vi "GOOP_LVClass_CreateNewWizard_Invoke.vi"(10 "New Item Parent":T1, 11 "Wizard":u64) -> (3 "Canceled":bool)   [LabVIEW 2020]
uses:
  <resource>/Framework/Providers/API/mxLvNIIM.ctl
  <resource>/Framework/Providers/Open_GDS/ClassProviders/Provider_EndevoGOOP300/GOOP300_SubVIs/GOOP300_MethodScopeType.ctl
  <resource>/Framework/Providers/Open_GDS/SubVIs/GOOP_ClassProviderClassType.ctl
  <resource>/Framework/Providers/Open_GDS/ClassProviders/Provider_BaseClassInterface/ClassWriter_class/ClassWriter.lvclass
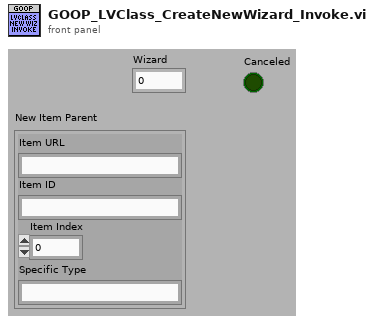
[diagram p1: front panel]
types:
  T1 = typedef "mxLvNIIM.ctl" = cluster{"Item URL":string, "Item ID":string, "Item Index":i32, "Specific Type":string}
  T2 = typedef "GOOP300_MethodScopeType.ctl" = enum16{"Use Parent Folder Scope", "Public", "Protected", "Private", "Community"}
  T3 = typedef "GOOP_ClassProviderClassType.ctl" = enum16{"ClassWriter", "ClassReader"}
  T4 = typedef "ClassWriter.lvclass/CreateClassData.ctl" = cluster{"ClassName":string, "ClassFolder":path, "ClassDescription":string, "ClassTemplateOptions":string, "BaseClass(ProjectStringPath or LvClassFilePath)":variant, "ExtraCreateParameters":variant, "FolderSuffix":string}
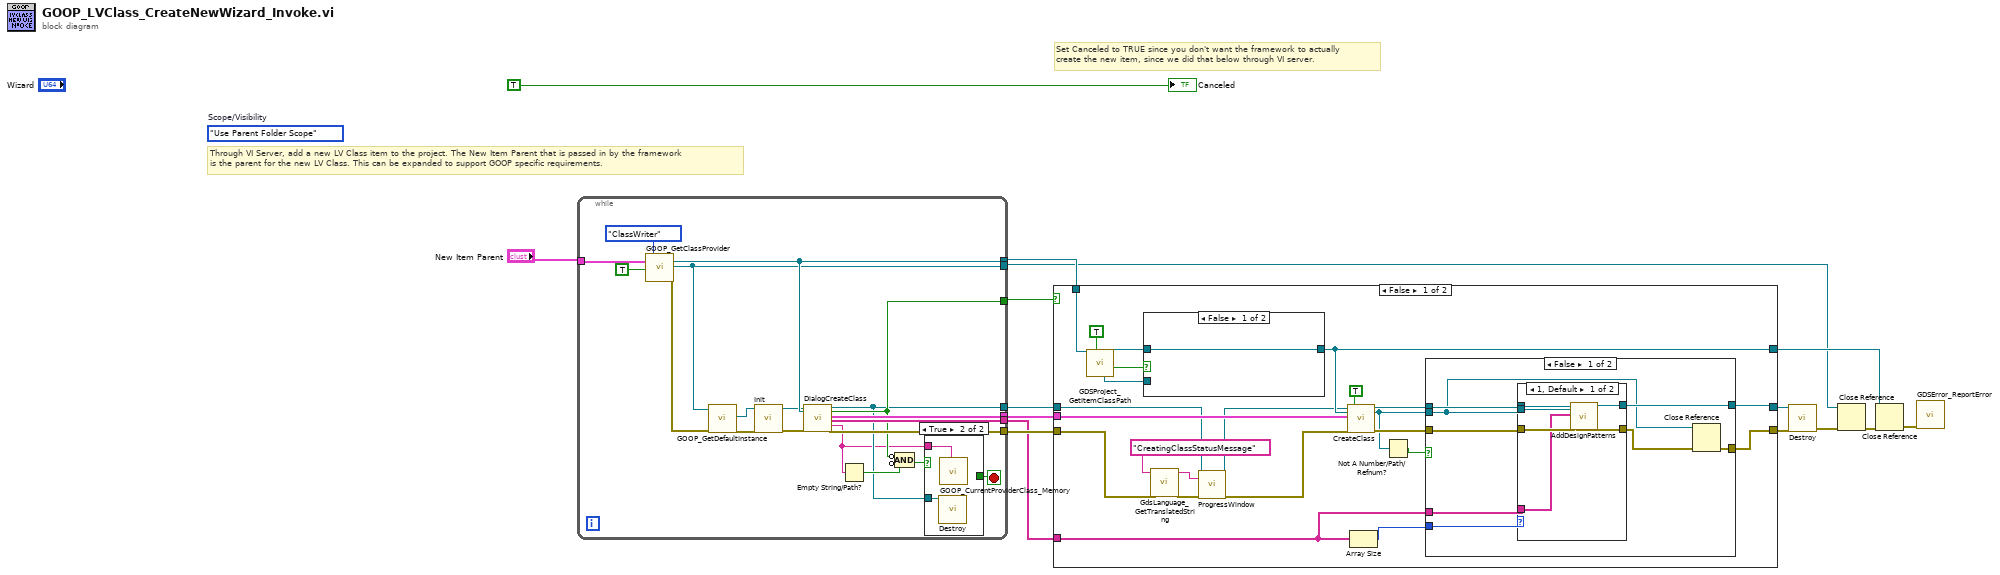
[diagram p0: block diagram]
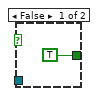
[diagram p2: hidden frame]
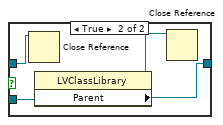
[diagram p5: hidden frame]
diagram:
  (unwired) GOOP300_MethodScopeType."Use Parent Folder Scope"  # Scope/Visibility
  # "Through VI Server, add a new LV Class item to the project. The New Item Parent that is passed in by the framework\nis the parent for the new LV Class. This can be expanded to support GOOP specific requirements."
  # "Set Canceled to TRUE since you don't want the framework to actually\ncreate the new item, since we did that below through VI server."
  n1 = while {
    tunnel: "New Item Parent" -> [w34]
    tunnel: [w17] -> w11
    tunnel: [w33] -> w10
    tunnel: [w32] -> w9
    tunnel: [w30] -> w6
    tunnel: [w25] -> w3
    tunnel: [w22] -> w2
    tunnel: [w21] -> w1
    stop <- w18 stop-if-true
    n2 = call <resource>:"GOOP_GetClassProvider.vi"("New Item Parent/Object"=w34, "CreateClass"=TRUE, "ProviderClassType"=GOOP_ClassProviderClassType."ClassWriter") -> ("ProjectItem"=w30:refnum<vi>, "LVClass.Open"=w25:refnum<vi>, "error out"=w24:errorcluster)  [unwired: 14 in]
    n3 = call <resource>:"GOOP_GetDefaultInstance.vi"("error in"=w24, "LVClassIn"=w25) -> ("error out"=w26:errorcluster, "ClassWriter.lvclass"=w23:refnum<class "ClassWriter.lvclass">)  [unwired: 7 in, 1 out]
    n4 = call-dynamic "Init.vi"("ClassWriter in"=w23, "error in (no error)"=w26) -> ("ClassWriter out"=w28:refnum<class "ClassWriter.lvclass">, "error out"=w27:errorcluster)  [unwired: 16 in]
    n5 = call-dynamic "DialogCreateClass.vi"("ClassWriter in"=w28, "ProjectItem Refnum"=w30, "error in (no error)"=w27) -> ("ClassWriter out"=w17:refnum<class "ClassWriter.lvclass">, "Cancelled"=w21:bool, "CreateClassData"=w32:T4, "DesignPatternsToAddAfterCreation"=w22:string[], "ChangeProviderRequested"=w16:string, "error out"=w33:errorcluster)  [unwired: 11 in]
    n6 = Empty String/Path?(string/path=w16) -> (empty?=w20:bool)
    n7 = Compound Arithmetic op=AND(invert w21, invert w20) -> (w19:bool)
    n8 = case shown="True" w19 {
      tunnel: w16 -> [_ w37]
      tunnel: [TRUE _] -> w18
      tunnel: w17 -> [_ w36]
      frame False {
      }
      frame True {
        n9 = call-dynamic "Destroy.vi"("ClassWriter.lvclass"=w36) -> ()  [unwired: 18 in, 1 out]
        n10 = call <resource>:"GOOP_CurrentProviderClass_Memory.vi"("SetDefaultClassProvider(Ignored if not wired)"=w37) -> ()  [unwired: 14 in, 5 out]
      }
    }
  }
  n11 = case shown="False" w1 {
    tunnel: [w40 w86] -> w14
    tunnel: [w48 w85] -> w13
    tunnel: w11 -> [w51 w86]
    tunnel: w10 -> [w45 w85]
    tunnel: w9 -> [w60 _]
    tunnel: w6 -> [w59 w84]
    tunnel: [w55 w84] -> w5
    tunnel: w2 -> [w44 _]
    frame False {
      n12 = call <resource>:"GDSProject_GetItemClassPath.vi"("ReturnRefToClass(False)"=TRUE, "ProjectItemRefIn"=w59) -> ("LvCLassFound"=w57:bool, "ProjectItemRefOut"=w56:refnum<vi>, "LvClassRef"=w54:refnum<vi>)  [unwired: 4 in, 3 out]
      n13 = case shown="False" w57 {
        tunnel: w56 -> [w79 w83]
        tunnel: [w79 w81] -> w55
        tunnel: w54 -> [_ w82]
        frame False {
        }
        frame True {
          n14 = Close Reference(reference=w83) -> ()  [unwired: 1 in, 1 out]
          n15 = property class="LVClassLibrary"(reference=w82) -> (reference out=w80:refnum<vi>, "Parent"=w81:refnum<vi>)  [unwired: 1 in, 1 out]
          n16 = Close Reference(reference=w80) -> ()  [unwired: 1 in, 1 out]
        }
      }
      n17 = call <resource>:"GdsLanguage_GetTranslatedString.vi"("StringID(s)"="CreatingClassStatusMessage" ("Message(Exit)"), "error in (no error)"=w45) -> ("FirstStringOut"=w53:string, "error out"=w46:errorcluster)  [unwired: 14 in, 2 out]
      n18 = call-dynamic "ProgressWindow.vi"("ClassWriter in"=w51, "Message(Exit)"=w53, "error in (no error)"=w46) -> ("ClassWriter out"=w50:refnum<class "ClassWriter.lvclass">, "error out"=w47:errorcluster)  [unwired: 15 in]
      n19 = call-dynamic "CreateClass.vi"("ClassWriter.lvclass"=w50, "ProjectTreePosition(String or Project Item Ref)"=w55, "CreateClassData"=w60, "error in (no error)"=w47, "KeepLvClassRefOpen(False)"=TRUE) -> ("ClassWriter.lvclass"=w42:refnum<class "ClassWriter.lvclass">, "LVClassLibraryRefnum"=w39:refnum<vi>, "error out"=w41:errorcluster)  [unwired: 11 in, 1 out]
      n20 = Array Size(array=w44) -> (size(s)=w43:i32)
      n21 = Not A Number/Path/Refnum?(number/path/refnum=w39) -> (NaN/Path/Refnum?=w38:bool)
      n22 = case shown="False" w38 {
        tunnel: [w68 w78] -> w48
        tunnel: w44 -> [w67 _]
        tunnel: w43 -> [w66 _]
        tunnel: w42 -> [w65 w77]
        tunnel: w41 -> [w64 w78]
        tunnel: [w63 w77] -> w40
        tunnel: w39 -> [w61 _]
        frame False {
          n23 = case shown="1, Default" w66 {
            tunnel: w65 -> [w74 w76]
            tunnel: w64 -> [w73 w75]
            tunnel: [w72 w75] -> w62
            tunnel: [w71 w76] -> w63
            tunnel: w67 -> [w70 _]
            tunnel: w61 -> [w69 _]
            frame 1, Default {
              n24 = call-dynamic "AddDesignPatterns.vi"("ClassWriterNative"=w74, "ClassItemRefIn"=w69, "DesignPatterns"=w70, "error in (no error)"=w73) -> ("ClassWriterNative"=w71:refnum<class "ClassWriter.lvclass">, "error out"=w72:errorcluster)  [unwired: 12 in, 2 out]
            }
            frame 0 {
            }
          }
          n25 = Close Reference(reference=w61, error in (no error)=w62) -> (error out=w68:errorcluster)
        }
        frame True {
        }
      }
    }
    frame True {
    }
  }
  n26 = call-dynamic "Destroy.vi"("ClassWriter.lvclass"=w14, "error in (no error)"=w13) -> ("error out"=w8:errorcluster)  [unwired: 17 in]
  n27 = Close Reference(reference=w3, error in (no error)=w8) -> (error out=w7:errorcluster)
  n28 = Close Reference(reference=w5, error in (no error)=w7) -> (error out=w4:errorcluster)
  n29 = call <resource>:"GDSError_ReportError.vi"("error in (no error)"=w4) -> ()  [unwired: 18 in, 1 out]
  "Canceled" <- TRUE ("Canceled")
